vi "FFStopTimer.vi"   [LabVIEW 2015]
uses:
  TRANCON/DLL/lwlscdll.dll
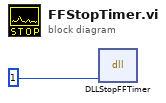
[diagram p0: block diagram]
diagram:
  n1 = dll-call lib="G:/SD/TRANCON/DLL/lwlscdll.dll" fn="DLLStopFFTimer"("drv"=u32 1) -> ()  [unwired: 5 in, 2 out]
